vi "CB Flywheel Moment of Intertia.vi"(9 "inner radius (in)":dbl, 10 "radius (in)":dbl, 11 "mass (lb)":dbl) -> (3 "moment of inertia":dbl)   [LabVIEW 2020]
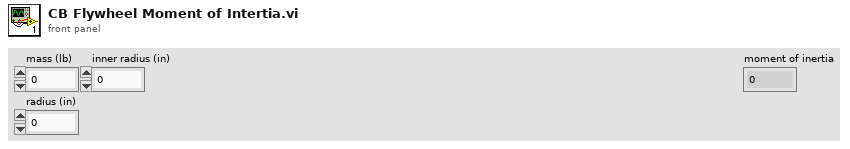
[diagram p1: front panel]
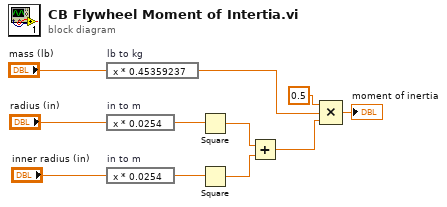
[diagram p0: block diagram]
diagram:
  n1 = expression code="x * 0.45359237" "lb to kg"("mass (lb)") -> (w4:dbl)
  n2 = expression code="x * 0.0254" "in to m"("radius (in)") -> (w8:dbl)
  n3 = expression code="x * 0.0254" "in to m"("inner radius (in)") -> (w7:dbl)
  n4 = Square(x=w8) -> (x^2=w6:dbl)
  n5 = Square(x=w7) -> (x^2=w5:dbl)
  n6 = Add(x=w6, y=w5) -> (x+y=w3:dbl)
  n7 = Compound Arithmetic op=MULTIPLY(0.5 ("value"), w4, w3) -> (→"moment of inertia":dbl)
